vi "Digital Signal.vi"(8 "error in (no error)":errorcluster caption="错误输入（无错误）", 9 "sample rate":dbl=1000.0 caption="采样率" format="%#_6p", 10 "number of signals":u32=8 caption="信号数", 11 "number of samples":u32=256 caption="采样数") -> (0 "error out":errorcluster caption="错误输出", 2 "digital waveform":digitalwaveform(waveform) caption="数字波形", 3 "数组":bool[][](array[boolean]))   [LabVIEW 2019]
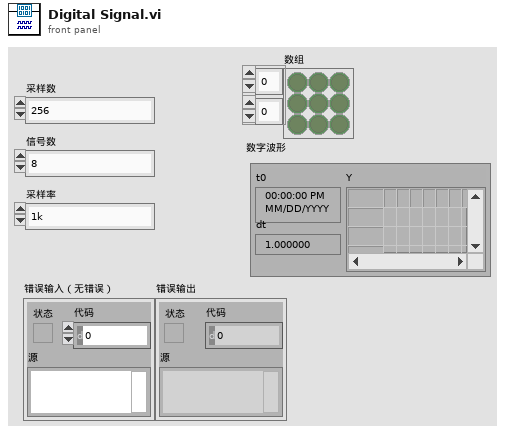
[diagram p1: front panel]
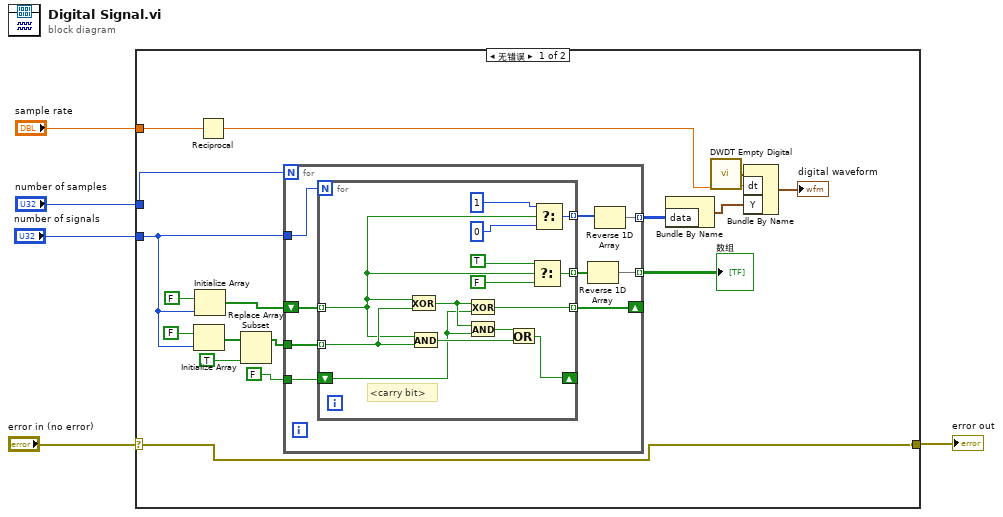
[diagram p0: block diagram]
diagram:
  n1 = case shown="无错误" "error in (no error)" {
    selector: "error in (no error)" -> [w12 w46]
    tunnel: [w12 w46] -> w4
    tunnel: "number of samples" -> [w14 _]
    tunnel: "sample rate" -> [w10 _]
    tunnel: "number of signals" -> [w15 _]
    frame No Error {
      n2 = Initialize Array(FALSE, w15) -> (w19:bool[])
      n3 = Initialize Array(FALSE, w15) -> (w21:bool[])
      n4 = Reciprocal(x=w10) -> (1/x=w7:dbl)
      n5 = Replace Array Subset(array=w19, new element=TRUE ("new element/subarray")) -> (w18:bool[])  [unwired: 1 in]
      n6 = for {
        N: w14 -> [_]
        tunnel: w15 -> [w31]
        shift-right: [w26] -> _
        shift-left: w21 -> [w28]
        tunnel: w18 -> [w30]
        tunnel: FALSE -> [w29]
        tunnel: [w25] -> w13 mode=indexing
        tunnel: [w23] -> w11 mode=indexing
        n7 = for {
          N: w31 -> [_]
          tunnel: w30 -> [w42] mode=indexing
          shift-right: [w40] -> _
          shift-left: w29 -> [w41]
          tunnel: w28 -> [w34] mode=indexing
          tunnel: [w38] -> w26 mode=indexing
          tunnel: [w39] -> w27 mode=indexing
          tunnel: [w32] -> w24 mode=indexing
          # "<carry bit>"
          n8 = Exclusive Or(1:w42, 2:w34) -> (0:w45:bool)
          n9 = And(x=w34, y=w42) -> (x .and. y?=w43:bool)
          n10 = Exclusive Or(1:w41, 2:w45) -> (0:w38:bool)
          n11 = And(x=w45, y=w41) -> (x .and. y?=w44:bool)
          n12 = Or(x=w44, y=w43) -> (x .or. y?=w40:bool)
          n13 = Select(t=TRUE, s=w34, f=FALSE) -> (s? t:f=w39:bool)
          n14 = Select(t=u8 1, s=w34, f=u8 0) -> (s? t:f=w32:u8)
        }
        n15 = Reverse 1D Array(array=w27) -> (reversed array=w25:bool[])
        n16 = Reverse 1D Array(array=w24) -> (reversed array=w23:u8[])
      }
      "数组" <- w13
      n17 = Bundle By Name("data"=w11) -> (w8:digitaldata)  [unwired: 1 in]
      n18 = call <vilib>:"DWDT Empty Digital.vi"() -> ("digital waveform out"=w9:digitalwaveform)  [unwired: 5 in]
      n19 = Bundle By Name(cluster=w9, "dt"=w7, "Y"=w8) -> (→"digital waveform":digitalwaveform)
    }
    frame Error {
    }
  }
  "error out" <- w4
